vi "InitializeGlobalSettings.vi"() -> (0 "Global Settings":T1)   [LabVIEW 2014]
uses:
  Controls/Global Settings/GlobalSettings.ctl
  Controls/Global Settings/InitialBackgroundValues.ctl
  Controls/Global Settings/GasPuffing.ctl
  Controls/Global Settings/PSUVoltages.ctl
  Controls/Global Settings/ScopeDetails.ctl
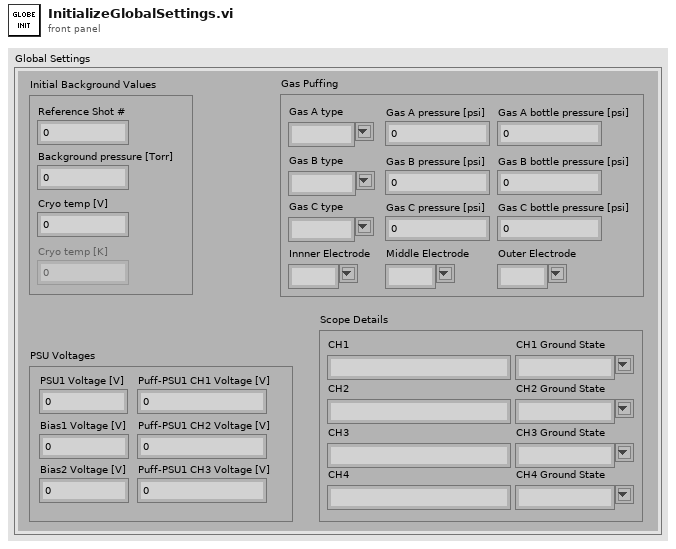
[diagram p1: front panel]
types:
  T1 = typedef "GlobalSettings.ctl" = cluster{"Initial Background Values":T2, "Gas Puffing":T3, "PSU Voltages":T4, "Scope Details":T5}
  T2 = typedef "InitialBackgroundValues.ctl" = cluster{"Reference Shot #":dbl, "Background pressure [Torr]":dbl, "Cryo temp [V]":dbl, "Cryo temp [K]":dbl}
  T3 = typedef "GasPuffing.ctl" = cluster{"Gas A type":string, "Gas B type":string, "Gas C type":string, "Gas A pressure [psi]":dbl, "Gas B pressure [psi]":dbl, "Gas C pressure [psi]":dbl, "Innner Electrode":string, "Middle Electrode":string, "Outer Electrode":string, "Gas A bottle pressure [psi]":dbl, "Gas B bottle pressure [psi]":dbl, "Gas C bottle pressure [psi]":dbl}
  T4 = typedef "PSUVoltages.ctl" = cluster{"Bias1 Voltage [V]":dbl, "Bias2 Voltage [V]":dbl, "PSU1 Voltage [V]":dbl, "Puff-PSU1 CH1 Voltage [V]":dbl, "Puff-PSU1 CH2 Voltage [V]":dbl, "Puff-PSU1 CH3 Voltage [V]":dbl}
  T5 = typedef "ScopeDetails.ctl" = cluster{"CH1":string, "CH2":string, "CH3":string, "CH4":string, "CH1 Ground State":string, "CH2 Ground State":string, "CH3 Ground State":string, "CH4 Ground State":string}
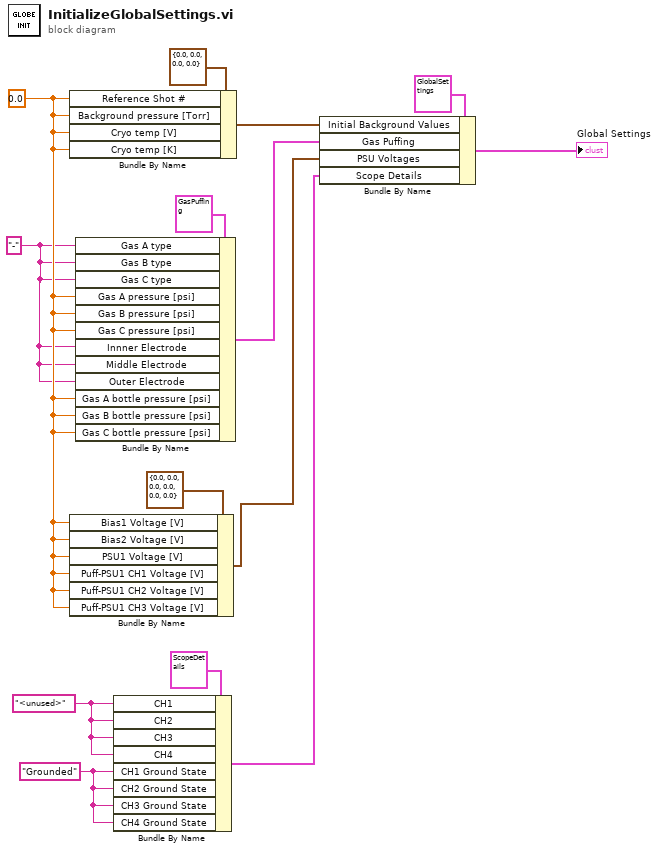
[diagram p0: block diagram]
diagram:
  w1 = "-" ("Innner Electrode")
  w2 = "Grounded" ("CH1 Ground State")
  w3 = "<unused>" ("CH1")
  w4 = 0.0 ("Cryo temp [V]")
  n1 = Bundle By Name(cluster=T2 {"Reference Shot #"=0.0, "Background pressure [Torr]"=0.0, "Cryo temp [V]"=0.0, "Cryo temp [K]"=0.0} ("Initial Background Values"), "Reference Shot #"=w4, "Background pressure [Torr]"=w4, "Cryo temp [V]"=w4, "Cryo temp [K]"=w4) -> (w8:T2)
  n2 = Bundle By Name(cluster=T4 {"Bias1 Voltage [V]"=0.0, "Bias2 Voltage [V]"=0.0, "PSU1 Voltage [V]"=0.0, "Puff-PSU1 CH1 Voltage [V]"=0.0, "Puff-PSU1 CH2 Voltage [V]"=0.0, "Puff-PSU1 CH3 Voltage [V]"=0.0} ("PSU Voltages"), "Bias1 Voltage [V]"=w4, "Bias2 Voltage [V]"=w4, "PSU1 Voltage [V]"=w4, "Puff-PSU1 CH1 Voltage [V]"=w4, "Puff-PSU1 CH2 Voltage [V]"=w4, "Puff-PSU1 CH3 Voltage [V]"=w4) -> (w12:T4)
  n3 = Bundle By Name(cluster=T3 {"Gas A type"="N", "Gas B type"="N", "Gas C type"="N", "Gas A pressure [psi]"=0.0, "Gas B pressure [psi]"=0.0, "Gas C pressure [psi]"=0.0, "Innner Electrode"="", "Middle Electrode"="", "Outer Electrode"="", "Gas A bottle pressure [psi]"=0.0, "Gas B bottle pressure [psi]"=0.0, "Gas C bottle pressure [psi]"=0.0} ("Gas Puffing"), "Gas A type"=w1, "Gas B type"=w1, "Gas C type"=w1, "Gas A pressure [psi]"=w4, "Gas B pressure [psi]"=w4, "Gas C pressure [psi]"=w4, "Innner Electrode"=w1, "Middle Electrode"=w1, "Outer Electrode"=w1, "Gas A bottle pressure [psi]"=w4, "Gas B bottle pressure [psi]"=w4, "Gas C bottle pressure [psi]"=w4) -> (w10:T3)
  n4 = Bundle By Name(cluster=T5 {"CH1"="", "CH2"="", "CH3"="", "CH4"="", "CH1 Ground State"="Grounded", "CH2 Ground State"="Grounded", "CH3 Ground State"="Grounded", "CH4 Ground State"="Grounded"} ("Scope Details"), "CH1"=w3, "CH2"=w3, "CH3"=w3, "CH4"=w3, "CH1 Ground State"=w2, "CH2 Ground State"=w2, "CH3 Ground State"=w2, "CH4 Ground State"=w2) -> (w14:T5)
  n5 = Bundle By Name(cluster=T1 {"Initial Background Values"={"Reference Shot #"=0.0, "Background pressure [Torr]"=0.0, "Cryo temp [V]"=0.0, "Cryo temp [K]"=0.0}, "Gas Puffing"={"Gas A type"="N", "Gas B type"="N", "Gas C type"="N", "Gas A pressure [psi]"=0.0, "Gas B pressure [psi]"=0.0, "Gas C pressure [psi]"=0.0, "Innner Electrode"="", "Middle Electrode"="", "Outer Electrode"="", "Gas A bottle pressure [psi]"=0.0, "Gas B bottle pressure [psi]"=0.0, "Gas C bottle pressure [psi]"=0.0}, "PSU Voltages"={"Bias1 Voltage [V]"=0.0, "Bias2 Voltage [V]"=0.0, "PSU1 Voltage [V]"=0.0, "Puff-PSU1 CH1 Voltage [V]"=0.0, "Puff-PSU1 CH2 Voltage [V]"=0.0, "Puff-PSU1 CH3 Voltage [V]"=0.0}, "Scope Details"={"CH1"="", "CH2"="", "CH3"="", "CH4"="", "CH1 Ground State"="Grounded", "CH2 Ground State"="Grounded", "CH3 Ground State"="Grounded", "CH4 Ground State"="Grounded"}} ("Global Settings"), "Initial Background Values"=w8, "Gas Puffing"=w10, "PSU Voltages"=w12, "Scope Details"=w14) -> (→"Global Settings":T1)
